vi "simple tcp listener.vi"(4 "data":variant[](array[variant]), 6 "terminals":string[](array[string]), 9 "stop notification":refnum<notifier>, 10 "callback VI Refnum":refnum<vi>, 11 "port":u16) -> ()   [LabVIEW 2013, in "NISE Tools VI Server.lvlib"]
doc: "This VI acts as a TCP server."
uses:
  NISE Tools VI Server.lvlib
  run reference with parameters.vi
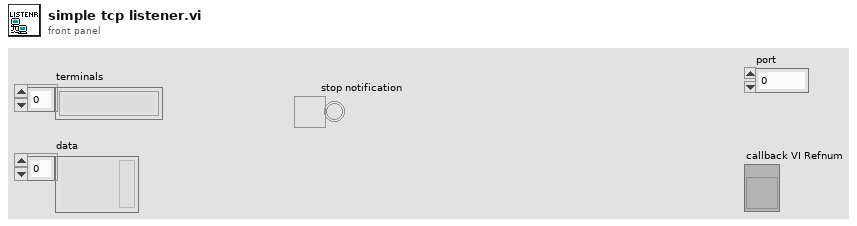
[diagram p1: front panel]
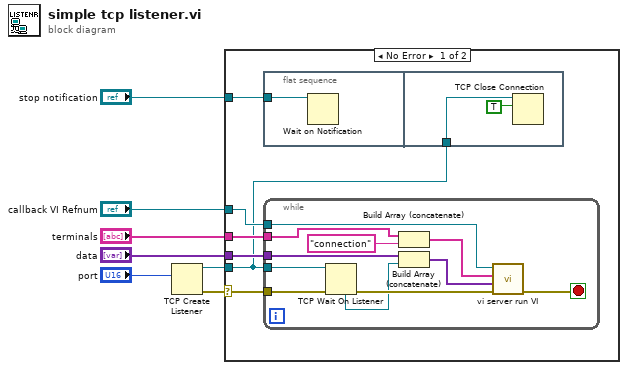
[diagram p0: block diagram]
diagram:
  n1 = TCP Create Listener(10:"port") -> (0:w6:errorcluster, 3:w5:refnum<k5>)  [unwired: 4 in, 1 out]
  n2 = case shown="No Error" w6 {
    selector: w6 -> [w13 _]
    tunnel: w5 -> [w8 _]
    tunnel: "callback VI Refnum" -> [w12 _]
    tunnel: "terminals" -> [w10 _]
    tunnel: "data" -> [w11 _]
    tunnel: "stop notification" -> [w9 _]
    frame No Error {
      n3 = flat-sequence {
        tunnel: w9 -> [w25]
        tunnel: w8 -> [w27]
        frame #0 {
          n4 = Wait on Notification(notifier=w25) -> ()  [unwired: 3 in, 4 out]
        }
        frame #1 {
          n5 = TCP Close Connection(connection ID=w27, abort (F)=TRUE) -> ()  [unwired: 1 in, 2 out]
        }
      }
      n6 = while {
        tunnel: w13 -> [w24]
        tunnel: w12 -> [w22]
        tunnel: w11 -> [w21]
        tunnel: w10 -> [w20]
        tunnel: w8 -> [w15]
        stop <- w14 stop-if-true
        n7 = TCP Wait On Listener(8:w24, 11:w15) -> (0:w23:errorcluster, 4:w17:refnum<k5>)  [unwired: 2 in, 3 out]
        n8 = Build Array (concatenate)(w20, "connection" ("String")) -> (w19:string[])
        n9 = Build Array (concatenate)(w21, w17) -> (w18:variant[])
        n10 = call-poly "vi server run VI.vi"("error in"=w23, "data"=w18, "terminals"=w19, "VI Refnum"=w22) -> ("error out"=w14:errorcluster)  [unwired: 7 in]
      }
    }
    frame Error {
    }
  }
